vi "make_stop_q.vi"(8 "error in (no error)":errorcluster) -> (0 "error out":errorcluster, 3 "stop_q":refnum<queue>)   [LabVIEW 2018]
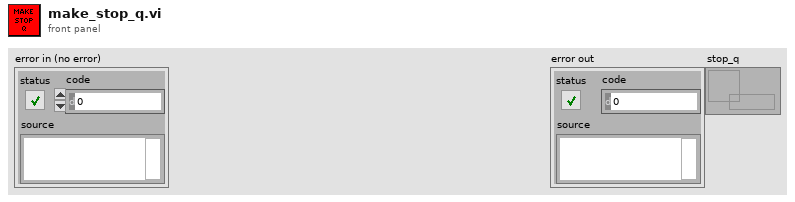
[diagram p1: front panel]
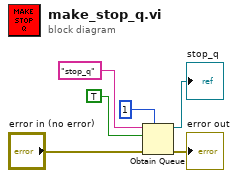
[diagram p0: block diagram]
diagram:
  n1 = Obtain Queue(max queue size (-1, unlimited)=1, name (unnamed)="stop_q", element data type=TRUE, error in (no error)="error in (no error)") -> (queue out=→"stop_q":refnum<queue>, error out=→"error out":errorcluster)  [unwired: 1 in, 1 out]
